vi "Gyro.vi"   [LabVIEW 2017]
uses:
  <vilib>/Rock Robotics/Network Tables/NT Read Boolean.vi
  <vilib>/Rock Robotics/Network Tables/NT Write Number.vi
types:
  T1 = typedef "WPI_GyroDevRef.ctl" = cluster{"DevStatus":errorcluster, "Analog Channel":T2, "Gain (VoltsPerDegree/Second)":dbl, "Gyro Type":enum16{"Analog", "XRS450"}, "Handle":i32, "SPI Bus":T3, "Device Found":bool, "Sample Rate":dbl, "Calibrate On Open":bool, "Offset":dbl}
  T2 = typedef "FPGA_AIChannel.ctl" = enum8{"AI 0", "AI 1", "AI 2", "AI 3", "AI MXP 0", "AI MXP 1", "AI MXP 2", "AI MXP 3", "Invalid"}
  T3 = typedef "spi_bus.ctl" = enum16{"SPI On-Board, CS0", "SPI On-Board, CS1", "SPI On-Board, CS2", "SPI On-Board, CS3", "SPI MXP", "Invalid"}
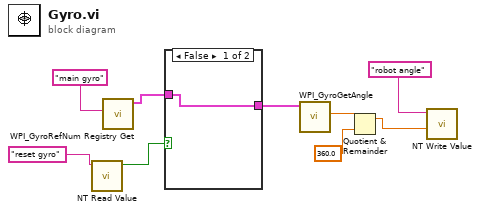
[diagram p0: block diagram]
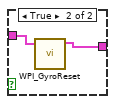
[diagram p2: hidden frame]
diagram:
  n1 = call-poly <vilib>:"NT Read Value.vi"("Name"="reset gyro") -> ("Boolean"=w8:bool)  [unwired: 9 in, 1 out]
  n2 = call <vilib>:"WPI_GyroRefNum Registry Get.vi"("refnum name"="main gyro") -> ("GyroDevRef"=w5:T1)  [unwired: 9 in, 1 out]
  n3 = case shown="False" w8 {
    tunnel: w5 -> [w10 w12]
    tunnel: [w10 w11] -> w6
    frame False {
    }
    frame True {
      n4 = call <vilib>:"WPI_GyroReset.vi"("GyroDevRef"=w12) -> ("GyroDevRef"=w11:T1)  [unwired: 9 in, 1 out]
    }
  }
  n5 = call <vilib>:"WPI_GyroGetAngle.vi"("GyroDevRef"=w6) -> ("Angle"=w7:dbl)  [unwired: 6 in, 4 out]
  n6 = Quotient & Remainder(x=w7, y=360.0) -> (x-y*floor(x/y)=w4:dbl)  [unwired: 1 out]
  n7 = call-poly <vilib>:"NT Write Value.vi"("Numeric"=w4, "Name"="robot angle") -> ()  [unwired: 9 in, 1 out]
